vi "Write Voltage.vi"(8 "error in":errorcluster, 10 "Voltage":dbl, 11 "36234A in":refnum<class "36234A.lvclass">) -> (0 "error out":errorcluster, 3 "36234A out":refnum<class "36234A.lvclass">)   [LabVIEW 2019, in "36234A.lvlib" / "36234A.lvclass"]
uses:
  Library/36234A.lvclass
  builds/Instruments/PowerSupply.lvlibp/Library/PowerSupply.lvclass
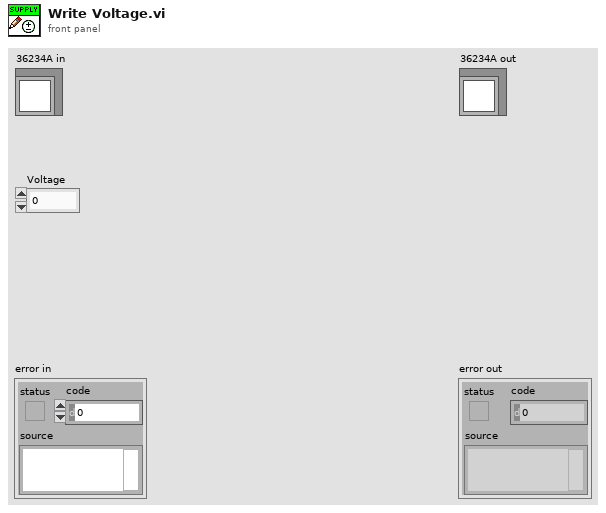
[diagram p1: front panel]
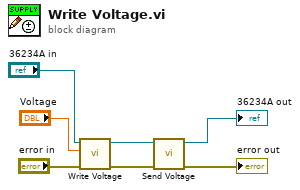
[diagram p0: block diagram]
diagram:
  n1 = call-parent "Write Voltage.vi"("error in"="error in", "Voltage"="Voltage", "PowerSupply in"="36234A in") -> ("error out"=w3:errorcluster, "PowerSupply out"=w4:refnum<class "36234A.lvclass">)  [unwired: 7 in]
  n2 = call "Send Voltage.vi"("error in (no error)"=w3, "36234A in"=w4) -> ("error out"=→"error out":errorcluster, "36234A out"=→"36234A out":refnum<class "36234A.lvclass">)  [unwired: 8 in]
